vi "JKISM++ Revert Arguments-Safe String.vi"(2 "Safe Argurment String":string="eaasdf->fqwvrf") -> (7 "Origin Argurment String":string)   [LabVIEW 2014, in "JKI State Machine++.lvlib"]
doc: "'->','->|','-@','-&','<-\" 是关键字，不能出现在参数中。使用<b>JKISM++ Make String Arguments Safe.vi</b>保证参数安全。此VI用于将安全参数转换为原始参数。\n\n<b>Inputs:</b>\n - <b>Safe Argurment String</b>: 安全参数\n\n<b>Outputs:</b>\n - <b>Origin Argurment String</b>: 可能包含关键字的参数 '->','->|','-@','-&','<-\"."
uses:
  JKI State Machine++.lvlib
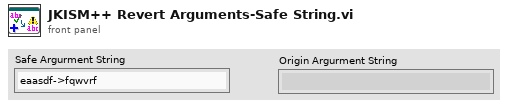
[diagram p1: front panel]
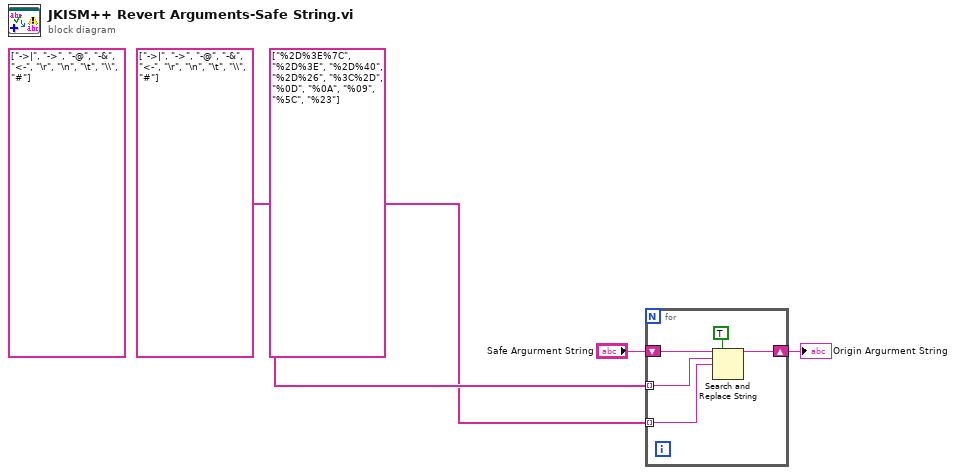
[diagram p0: block diagram]
diagram:
  (unwired) string[] ["->|", "->", "-@", "-&", "<-", "\r", "\n", "\t", "\\", "#"]
  n1 = for {
    shift-right: [w7] -> w3
    shift-left: "Safe Argurment String" -> [w9]
    tunnel: string[] ["->|", "->", "-@", "-&", "<-", "\r", "\n", "\t", "\\", "#"] -> [w6] mode=indexing
    tunnel: string[] ["%2D%3E%7C", "%2D%3E", "%2D%40", "%2D%26", "%3C%2D", "%0D", "%0A", "%09", "%5C", "%23"] -> [w5] mode=indexing
    n2 = Search and Replace String(replace all?=TRUE ("replace all? (F)"), input string=w9, search string=w6, replace string=w5) -> (result string=w7:string)  [unwired: 4 in, 3 out]
  }
  "Origin Argurment String" <- w3
